vi "UI_write_into_tdms.vi"(4 "beads info":T4[](array[typedef]), 6 "write mode":enum16{"XYZ", "XYZ_err", "Z"}(ring), 7 "Piezo":refnum<vi>, 8 "rec array输入":dbl[][][](array[numeric]), 9 "reference in":refnum<vi>, 10 "Public":T1 {"ROI descriptors"."Contours"."Type" items=["No Selection", "Point", "Line", "Rectangle", "Oval", "Polygon", "Freehand Region", "Annulus", "Unused2", "Unused3", "Broken Line", "Freehand Line", "Rotated Rectangle"]; "ROI Descriptor out"."Contours"."Type" items=["No Selection", "Point", "Line", "Rectangle", "Oval", "Polygon", "Freehand Region", "Annulus", "Unused2", "Unused3", "Broken Line", "Freehand Line", "Rotated Rectangle"]}, 11 "Digital in":refnum<vi>) -> ()   [LabVIEW 2017]
uses:
  control/bead info.ctl
  <vilib>/vision/Image Controls.llb/IMAQ Image.ctl
  control/beads public.ctl
  control/record mode.ctl
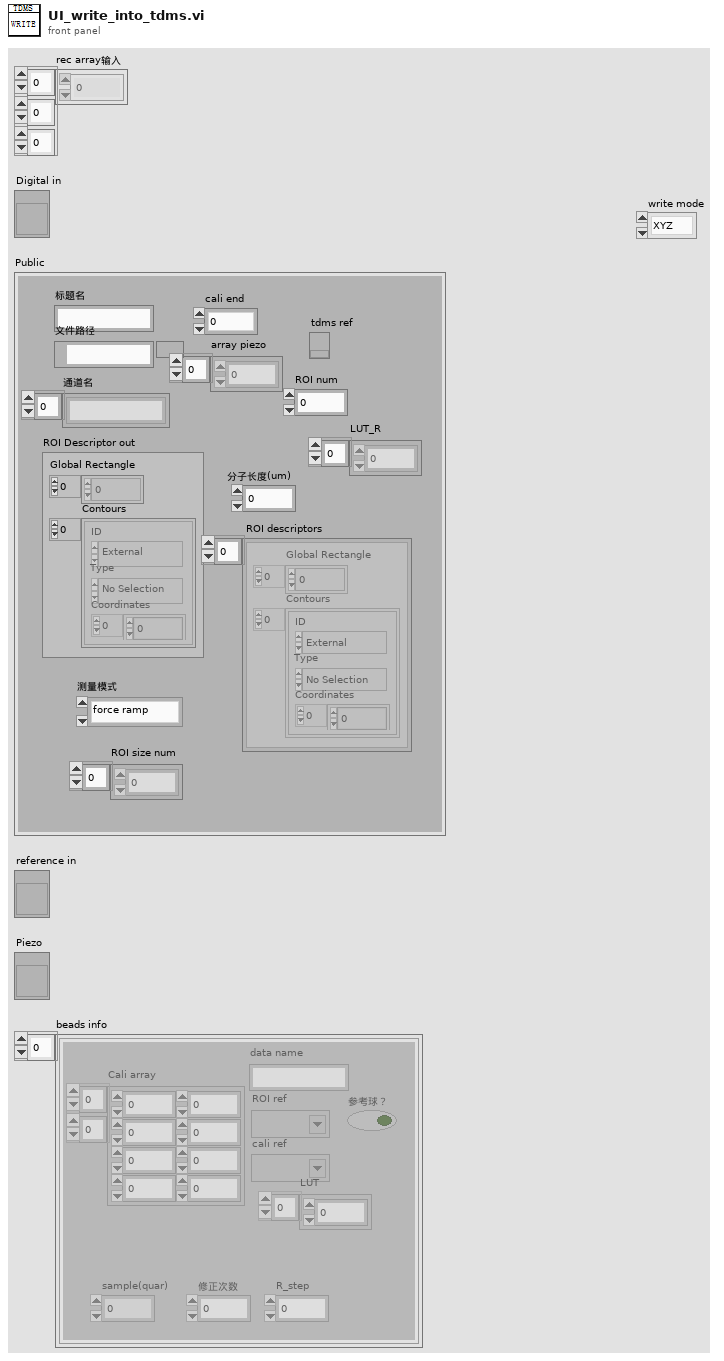
[diagram p1: front panel]
types:
  T1 = typedef "beads public.ctl" = cluster{"标题名":string, "文件路径":path, "通道名":string[], "ROI Descriptor out":T2, "cali end":dbl, "array piezo":dbl[], "LUT_R":dbl[], " ROI descriptors ":T2[], "tdms ref":refnum<k34>, "分子长度(um)":dbl, "ROI num":i32, "ROI size num":i32[], "测量模式":T3}
  T2 = typedef "ROI Descriptor" = cluster{"Global Rectangle":i32[], "Contours":cluster{"ID":enum32{"External", "Internal"}, "Type":u32, "Coordinates":i32[]}[]}
  T3 = typedef "record mode.ctl" = enum16{"force ramp", "force clamp", "force jump", "user-defined"}
  T4 = typedef "bead info.ctl" = cluster{"data name":string, "ROI ref":T5, "cali ref":T5, "参考球？":bool, "LUT":dbl[], "Cali array":dbl[][], "修正次数":i32, "R_step":dbl, "sample(quar)":i32}
  T5 = typedef "IMAQ Image.ctl" = refnum<image>
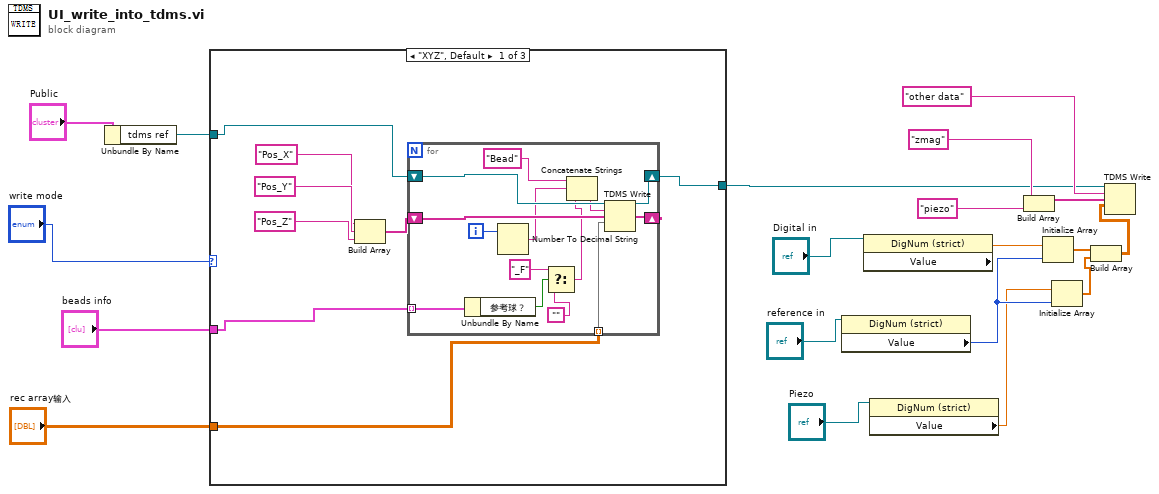
[diagram p0: block diagram]
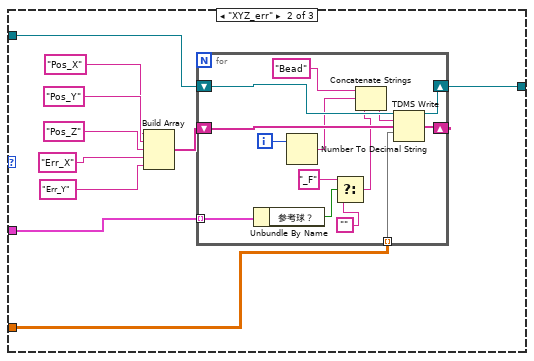
[diagram p2: hidden frame]
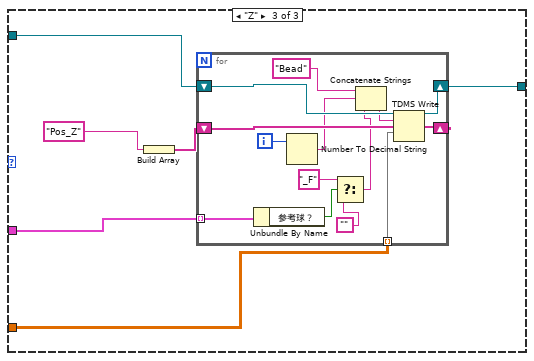
[diagram p3: hidden frame]
diagram:
  n1 = Unbundle By Name("Public") -> ("tdms ref"=w5:refnum<k34>)
  n2 = case shown="\"XYZ\", Default" "write mode" {
    tunnel: "rec array输入" -> [w21 w51 w71]
    tunnel: "beads info" -> [w22 w50 w70]
    tunnel: [w20 w49 w69] -> w7
    tunnel: w5 -> [w23 w44 w66]
    frame "XYZ", Default {
      n3 = Build Array("Pos_X" ("字符串"), "Pos_Y" ("字符串"), "Pos_Z" ("字符串")) -> (w27:string[])
      n4 = for {
        shift-right: [w35] -> w20
        shift-left: w23 -> [w41]
        shift-right: [w34] -> _
        shift-left: w27 -> [w40]
        tunnel: w21 -> [w33] mode=indexing
        tunnel: w22 -> [w32] mode=indexing
        i -> [w37]
        n5 = Unbundle By Name(w32) -> ("参考球？"=w31:bool)
        n6 = Number To Decimal String(number=w37) -> (decimal integer string=w36:string)  [unwired: 1 in]
        n7 = Select(t="_F", s=w31, f="") -> (s? t:f=w28:string)
        n8 = Concatenate Strings("Bead" ("字符串"), w36, w28) -> (w39:string)
        n9 = TDMS Write(0:w41, 5:w39, 7:w40, 9:w33) -> (4:w35:refnum<k34>, 8:w34:string[])  [unwired: 2 in, 2 out]
      }
    }
    frame "XYZ_err" {
      n10 = Build Array("Pos_X" ("字符串"), "Pos_Y" ("字符串"), "Pos_Z" ("字符串"), "Err_X" ("字符串"), "Err_Y" ("字符串")) -> (w48:string[])
      n11 = for {
        shift-right: [w59] -> w49
        shift-left: w44 -> [w65]
        shift-right: [w58] -> _
        shift-left: w48 -> [w64]
        tunnel: w51 -> [w57] mode=indexing
        tunnel: w50 -> [w56] mode=indexing
        i -> [w61]
        n12 = Unbundle By Name(w56) -> ("参考球？"=w55:bool)
        n13 = Number To Decimal String(number=w61) -> (decimal integer string=w60:string)  [unwired: 1 in]
        n14 = Select(t="_F", s=w55, f="") -> (s? t:f=w52:string)
        n15 = Concatenate Strings("Bead" ("字符串"), w60, w52) -> (w63:string)
        n16 = TDMS Write(0:w65, 5:w63, 7:w64, 9:w57) -> (4:w59:refnum<k34>, 8:w58:string[])  [unwired: 2 in, 2 out]
      }
    }
    frame "Z" {
      n17 = Build Array("Pos_Z" ("字符串")) -> (w68:string[])
      n18 = for {
        shift-right: [w79] -> w69
        shift-left: w66 -> [w85]
        shift-right: [w78] -> _
        shift-left: w68 -> [w84]
        tunnel: w71 -> [w77] mode=indexing
        tunnel: w70 -> [w76] mode=indexing
        i -> [w81]
        n19 = Unbundle By Name(w76) -> ("参考球？"=w75:bool)
        n20 = Number To Decimal String(number=w81) -> (decimal integer string=w80:string)  [unwired: 1 in]
        n21 = Select(t="_F", s=w75, f="") -> (s? t:f=w72:string)
        n22 = Concatenate Strings("Bead" ("字符串"), w80, w72) -> (w83:string)
        n23 = TDMS Write(0:w85, 5:w83, 7:w84, 9:w77) -> (4:w79:refnum<k34>, 8:w78:string[])  [unwired: 2 in, 2 out]
      }
    }
  }
  n24 = property class="DigNum (strict)"(reference="reference in") -> ("Value"=w14:i32)  [unwired: 1 in, 2 out]
  n25 = property class="DigNum (strict)"(reference="Digital in") -> ("Value"=w18:dbl)  [unwired: 1 in, 2 out]
  n26 = property class="DigNum (strict)"(reference="Piezo") -> ("Value"=w13:dbl)  [unwired: 1 in, 2 out]
  n27 = Build Array("zmag" ("组名称输入（无标题）"), "piezo" ("元素")) -> (w11:string[])
  n28 = Initialize Array(w18, w14) -> (w15:dbl[])
  n29 = Initialize Array(w13, w14) -> (w16:dbl[])
  n30 = Build Array(w15, w16) -> (w17:dbl[][])
  n31 = TDMS Write(0:w7, 5:"other data" ("组名称输入（无标题）"), 7:w11, 9:w17) -> ()  [unwired: 2 in, 4 out]
